vi "HP34970A Trigger.vi"(7 "error in (no error)":errorcluster, 9 "Command (0:Rem Trig)":T1(ring), 10 "VISA session":refnum<visa-resource-name>) -> (0 "error out":errorcluster, 3 "dup VISA session":refnum<visa-resource-name>)   [LabVIEW 2020]
doc: "This VI lets you trigger the instrument remotely (from your computer), place the instrument in \"wait for trigger\" state, or abort the scan."
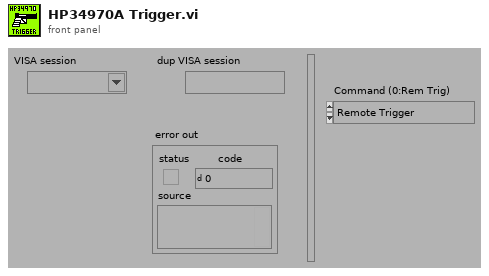
[diagram p1: front panel]
types:
  T1 = enum16{"Remote Trigger", "Immediate Trigger", "Wait for Trigger", "Abort Scan"}
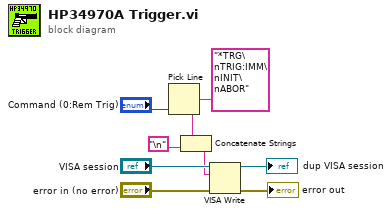
[diagram p0: block diagram]
diagram:
  n1 = Pick Line(multi-line string="*TRG\nTRIG:IMM\nINIT\nABOR", line index="Command (0:Rem Trig)") -> (output string=w3:string)  [unwired: 1 in]
  n2 = Concatenate Strings(w3, "\n") -> (w6:string)
  n3 = VISA Write(VISA resource name="VISA session", write buffer=w6, error in (no error)="error in (no error)") -> (VISA resource name out=→"dup VISA session":refnum<visa-resource-name>, error out=→"error out":errorcluster)  [unwired: 1 out]
